vi "rsidr_core_global.vi"() -> ()   [LabVIEW 2015, in "Rohde&Schwarz CMXP NR FR2 Measurement.lvlib"] (continued)
  in  "Range Tables":T3(array[cluster])=[{"Name"="rsCmxpNrFr2M_rngInputConnector", "Type"=enum."Discrete", "Entries"=[{"Name"="RF1COM", "Discrete or Min"=1.0, "Max"=0.0, "Coerced"=0.0, "Command"="\"P1.RRH.RF1\""}, {"Name"="RF2COM", "Discrete or Min"=2.0, "Max"=0.0, "Coerced"=0.0, "Command"="\"P1.RRH.RF2\""}, {"Name"="RF3COM", "Discrete or Min"=3.0, "Max"=0.0, "Coerced"=0.0, "Command"="\"P2.RRH.RF1\""}, {"Name"="RF4COM", "Discrete or Min"=4.0, "Max"=0.0, "Coerced"=0.0, "Command"="\"P2.RRH.RF2\""}, {"Name"="RF5COM", "Discrete or Min"=5.0, "Max"=0.0, "Coerced"=0.0, "Command"="\"P3.RRH.RF1\""}, {"Name"="RF6COM", "Discrete or Min"=6.0, "Max"=0.0, "Coerced"=0.0, "Command"="\"P3.RRH.RF2\""}, {"Name"="IF1IN", "Discrete or Min"=7.0, "Max"=0.0, "Coerced"=0.0, "Command"="\"P1.IFIn\""}, {"Name"="IF2IN", "Discrete or Min"=8.0, "Max"=0.0, "Coerced"=0.0, "Command"="\"P2.IFIn\""}, {"Name"="IF3IN", "Discrete or Min"=9.0, "Max"=0.0, "Coerced"=0.0, "Command"="\"P3.IFIn\""}]}, {"Name"="rsCmxpNrFr2M_rngExtAtt", "Type"=enum."Range", "Entries"=[{"Name"="", "Discrete or Min"=-50.0, "Max"=90.0, "Coerced"=0.0, "Command"=""}]}, {"Name"="rsCmxpNrFr2M_rngRepMode", "Type"=enum."Discrete", "Entries"=[{"Name"="Single shot measurement", "Discrete or Min"=0.0, "Max"=0.0, "Coerced"=0.0, "Command"="SING"}, {"Name"="Continuous measurement", "Discrete or Min"=1.0, "Max"=0.0, "Coerced"=0.0, "Command"="CONT"}]}, {"Name"="rsCmxpNrFr2M_rngStatCount", "Type"=enum."Range", "Entries"=[{"Name"="", "Discrete or Min"=1.0, "Max"=1000.0, "Coerced"=0.0, "Command"=""}]}, {"Name"="rsCmxpNrFr2M_rngTrigThreshold", "Type"=enum."Range", "Entries"=[{"Name"="", "Discrete or Min"=-50.0, "Max"=0.0, "Coerced"=0.0, "Command"=""}]}, {"Name"="rsCmxpNrFr2M_rngStopCondition", "Type"=enum."Discrete", "Entries"=[{"Name"="None", "Discrete or Min"=0.0, "Max"=0.0, "Coerced"=0.0, "Command"="NONE"}, {"Name"="Limit Failure", "Discrete or Min"=1.0, "Max"=0.0, "Coerced"=0.0, "Command"="SLF"}]}, {"Name"="rsCmxpNrFr2M_rngTrigSlope", "Type"=enum."Discrete", "Entries"=[{"Name"="Rising edge", "Discrete or Min"=0.0, "Max"=0.0, "Coerced"=0.0, "Command"="REDG"}, {"Name"="Falling Edge", "Discrete or Min"=1.0, "Max"=0.0, "Coerced"=0.0, "Command"="FEDG"}]}, {"Name"="rsCmxpNrFr2M_rngAnalyzerMixerLevelOffset", "Type"=enum."Range", "Entries"=[{"Name"="", "Discrete or Min"=-10.0, "Max"=10.0, "Coerced"=0.0, "Command"=""}]}, {"Name"="rsCmxpNrFr2M_rngInputSignalFrequencyBand", "Type"=enum."Discrete", "Entries"=[{"Name"="Band n257", "Discrete or Min"=0.0, "Max"=0.0, "Coerced"=0.0, "Command"="B257"}, {"Name"="Band n258", "Discrete or Min"=1.0, "Max"=0.0, "Coerced"=0.0, "Command"="B258"}, {"Name"="Band n260", "Discrete or Min"=2.0, "Max"=0.0, "Coerced"=0.0, "Command"="B260"}, {"Name"="Band n261", "Discrete or Min"=3.0, "Max"=0.0, "Coerced"=0.0, "Command"="B261"}]}, {"Name"="rsCmxpNrFr2M_rngAnalyzerFrequencyOffset", "Type"=enum."Range", "Entries"=[{"Name"="", "Discrete or Min"=-100000.0, "Max"=100000.0, "Coerced"=0.0, "Command"=""}]}, {"Name"="rsCmxpNrFr2M_rngMeasurementMode", "Type"=enum."Discrete", "Entries"=[{"Name"="Normal", "Discrete or Min"=0.0, "Max"=0.0, "Coerced"=0.0, "Command"="NORM"}, {"Name"="List Mode", "Discrete or Min"=1.0, "Max"=0.0, "Coerced"=0.0, "Command"="MELM"}]}, {"Name"="rsCmxpNrFr2M_rngListBand", "Type"=enum."Discrete", "Entries"=[{"Name"="B257", "Discrete or Min"=0.0, "Max"=0.0, "Coerced"=0.0, "Command"="B257"}, {"Name"="B258", "Discrete or Min"=1.0, "Max"=0.0, "Coerced"=0.0, "Command"="B258"}, {"Name"="B260", "Discrete or Min"=2.0, "Max"=0.0, "Coerced"=0.0, "Command"="B260"}, {"Name"="B261", "Discrete or Min"=3.0, "Max"=0.0, "Coerced"=0.0, "Command"="B261"}]}, {"Name"="rsCmxpNrFr2M_rngModScheme", "Type"=enum."Discrete", "Entries"=[{"Name"="Pi/2-BPSK", "Discrete or Min"=0.0, "Max"=0.0, "Coerced"=0.0, "Command"="PHBP"}, {"Name"="QPSK", "Discrete or Min"=1.0, "Max"=0.0, "Coerced"=0.0, "Command"="QPSK"}, {"Name"="16-QAM", "Discrete or Min"=2.0, "Max"=0.0, "Coerced"=0.0, "Command"="Q16"}, {"Name"="64-QAM", "Discrete or Min"=3.0, "Max"=0.0, "Coerced"=0.0, "Command"="Q64"}, {"Name"="256-QAM", "Discrete or Min"=4.0, "Max"=0.0, "Coerced"=0.0, "Command"="Q256"}]}, {"Name"="rsCmxpNrFr2M_rngOBWLimit", "Type"=enum."Range", "Entries"=[{"Name"="", "Discrete or Min"=0.0, "Max"=400000000.0, "Coerced"=0.0, "Command"=""}]}, {"Name"="rsCmxpNrFr2M_rngPhaseComp", "Type"=enum."Discrete", "Entries"=[{"Name"="Off", "Discrete or Min"=0.0, "Max"=0.0, "Coerced"=0.0, "Command"="OFF"}, {"Name"="Carrier Freq", "Discrete or Min"=1.0, "Max"=0.0, "Coerced"=0.0, "Command"="CAF"}, {"Name"="User Defined", "Discrete or Min"=2.0, "Max"=0.0, "Coerced"=0.0, "Command"="UDEF"}]}, {"Name"="rsCmxpNrFr2M_rngPUSCHMappingType", "Type"=enum."Discrete", "Entries"=[{"Name"="A", "Discrete or Min"=0.0, "Max"=0.0, "Coerced"=0.0, "Command"="A"}, {"Name"="B", "Discrete or Min"=1.0, "Max"=0.0, "Coerced"=0.0, "Command"="B"}]}, {"Name"="rsCmxpNrFr2M_rngPhysicalCellID", "Type"=enum."Range", "Entries"=[{"Name"="", "Discrete or Min"=0.0, "Max"=1007.0, "Coerced"=0.0, "Command"=""}]}, {"Name"="rsCmxpNrFr2M_rngTypeAPosition", "Type"=enum."Range", "Entries"=[{"Name"="", "Discrete or Min"=2.0, "Max"=3.0, "Coerced"=0.0, "Command"=""}]}, {"Name"="rsCmxpNrFr2M_rngTriggerTimeout", "Type"=enum."Range", "Entries"=[{"Name"="", "Discrete or Min"=0.01, "Max"=167772.15, "Coerced"=0.0, "Command"=""}]}, {"Name"="rsCmxpNrFr2M_rngResultType", "Type"=enum."Discrete", "Entries"=[{"Name"="Current", "Discrete or Min"=0.0, "Max"=0.0, "Coerced"=0.0, "Command"="CURR"}, {"Name"="Average", "Discrete or Min"=1.0, "Max"=0.0, "Coerced"=0.0, "Command"="AVER"}, {"Name"="Extreme", "Discrete or Min"=2.0, "Max"=0.0, "Coerced"=0.0, "Command"="EXTR"}, {"Name"="Standard Deviation", "Discrete or Min"=3.0, "Max"=0.0, "Coerced"=0.0, "Command"="SDEV"}, {"Name"="Maximum", "Discrete or Min"=4.0, "Max"=0.0, "Coerced"=0.0, "Command"="MAX"}, {"Name"="Minimum", "Discrete or Min"=5.0, "Max"=0.0, "Coerced"=0.0, "Command"="MIN"}]}, {"Name"="rsCmxpNrFr2M_rngWindowPosition", "Type"=enum."Discrete", "Entries"=[{"Name"="Low", "Discrete or Min"=0.0, "Max"=0.0, "Coerced"=0.0, "Command"="LOW"}, {"Name"="High", "Discrete or Min"=1.0, "Max"=0.0, "Coerced"=0.0, "Command"="HIGH"}]}, {"Name"="rsCmxpNrFr2M_rngPosNeg", "Type"=enum."Discrete", "Entries"=[{"Name"="Negative", "Discrete or Min"=0.0, "Max"=0.0, "Coerced"=0.0, "Command"="NEG"}, {"Name"="Positive", "Discrete or Min"=1.0, "Max"=0.0, "Coerced"=0.0, "Command"="POS"}]}, {"Name"="rsCmxpNrFr2M_rngMaxMin", "Type"=enum."Discrete", "Entries"=[{"Name"="Minimum", "Discrete or Min"=0.0, "Max"=0.0, "Coerced"=0.0, "Command"="MIN"}, {"Name"="Maximum", "Discrete or Min"=1.0, "Max"=0.0, "Coerced"=0.0, "Command"="MAX"}]}, {"Name"="rsCmxpNrFr2M_rngLowHigh", "Type"=enum."Discrete", "Entries"=[{"Name"="Low", "Discrete or Min"=0.0, "Max"=0.0, "Coerced"=0.0, "Command"="LOW"}, {"Name"="High", "Discrete or Min"=1.0, "Max"=0.0, "Coerced"=0.0, "Command"="HIGH"}]}, {"Name"="rsCmxpNrFr2M_rngPeriodicity", "Type"=enum."Discrete", "Entries"=[{"Name"="0.5 ms", "Discrete or Min"=0.0, "Max"=0.0, "Coerced"=0.0, "Command"="MS05"}, {"Name"="0.625 ms", "Discrete or Min"=1.0, "Max"=0.0, "Coerced"=0.0, "Command"="MS0625"}, {"Name"="1 ms", "Discrete or Min"=2.0, "Max"=0.0, "Coerced"=0.0, "Command"="MS1"}, {"Name"="1.25 ms", "Discrete or Min"=3.0, "Max"=0.0, "Coerced"=0.0, "Command"="MS125"}, {"Name"="2 ms", "Discrete or Min"=4.0, "Max"=0.0, "Coerced"=0.0, "Command"="MS2"}, {"Name"="2.5 ms", "Discrete or Min"=5.0, "Max"=0.0, "Coerced"=0.0, "Command"="MS25"}, {"Name"="5 ms", "Discrete or Min"=6.0, "Max"=0.0, "Coerced"=0.0, "Command"="MS5"}, {"Name"="10 ms", "Discrete or Min"=7.0, "Max"=0.0, "Coerced"=0.0, "Command"="MS10"}]}, {"Name"="rsCmxpNrFr2M_rngSubcarrierSpacing", "Type"=enum."Discrete", "Entries"=[{"Name"="60 kHz", "Discrete or Min"=0.0, "Max"=0.0, "Coerced"=0.0, "Command"="S60K"}, {"Name"="120 kHz", "Discrete or Min"=1.0, "Max"=0.0, "Coerced"=0.0, "Command"="S120"}]}, {"Name"="rsCmxpNrFr2M_rngChannelBandwidth", "Type"=enum."Discrete", "Entries"=[{"Name"="50 MHz", "Discrete or Min"=0.0, "Max"=0.0, "Coerced"=0.0, "Command"="B050"}, {"Name"="100 MHz", "Discrete or Min"=1.0, "Max"=0.0, "Coerced"=0.0, "Command"="B100"}, {"Name"="200 MHz", "Discrete or Min"=2.0, "Max"=0.0, "Coerced"=0.0, "Command"="B200"}, {"Name"="400 MHz", "Discrete or Min"=3.0, "Max"=0.0, "Coerced"=0.0, "Command"="B400"}]}, {"Name"="rsCmxpNrFr2M_rngDMRSSequenceGenerationUsedID", "Type"=enum."Discrete", "Entries"=[{"Name"="Cell ID Used", "Discrete or Min"=0.0, "Max"=0.0, "Coerced"=0.0, "Command"="CID"}, {"Name"="DMRS ID Used", "Discrete or Min"=1.0, "Max"=0.0, "Coerced"=0.0, "Command"="DMRS"}]}, {"Name"="rsCmxpNrFr2M_rngBandwidthFrequency", "Type"=enum."Discrete", "Entries"=[{"Name"="50 MHz", "Discrete or Min"=0.0, "Max"=0.0, "Coerced"=0.0, "Command"="50"}, {"Name"="100 MHz", "Discrete or Min"=1.0, "Max"=0.0, "Coerced"=0.0, "Command"="100"}, {"Name"="200 MHz", "Discrete or Min"=2.0, "Max"=0.0, "Coerced"=0.0, "Command"="200"}, {"Name"="400 MHz", "Discrete or Min"=3.0, "Max"=0.0, "Coerced"=0.0, "Command"="400"}]}, {"Name"="rsCmxpNrFr2M_rngMultiEvalMeasurementSpectrumMeasFilter", "Type"=enum."Discrete", "Entries"=[{"Name"="Bandpass", "Discrete or Min"=0.0, "Max"=0.0, "Coerced"=0.0, "Command"="BAND"}, {"Name"="Gauss", "Discrete or Min"=1.0, "Max"=0.0, "Coerced"=0.0, "Command"="GAUS"}]}, {"Name"="rsCmxpNrFr2M_rngMultiEvalMeasurementTriggerDelay", "Type"=enum."Range", "Entries"=[{"Name"="", "Discrete or Min"=-0.00025, "Max"=0.00025, "Coerced"=0.0, "Command"=""}]}, {"Name"="rsCmxpNrFr2M_rngMultiEvalMeasurementMinimumTriggerGap", "Type"=enum."Range", "Entries"=[{"Name"="", "Discrete or Min"=0.0, "Max"=0.001, "Coerced"=0.0, "Command"=""}]}, {"Name"="rsCmxpNrFr2M_rngRetriggerFlag", "Type"=enum."Discrete", "Entries"=[{"Name"="Off", "Discrete or Min"=0.0, "Max"=0.0, "Coerced"=0.0, "Command"="OFF"}, {"Name"="On", "Discrete or Min"=1.0, "Max"=0.0, "Coerced"=0.0, "Command"="ON"}, {"Name"="IF Power", "Discrete or Min"=2.0, "Max"=0.0, "Coerced"=0.0, "Command"="IFP"}]}, {"Name"="rsCmxpNrFr2M_rngLimitEnabled", "Type"=enum."Discrete", "Entries"=[{"Name"="Off", "Discrete or Min"=0.0, "Max"=0.0, "Coerced"=0.0, "Command"="OFF"}, {"Name"="On", "Discrete or Min"=1.0, "Max"=0.0, "Coerced"=0.0, "Command"="ON"}, {"Name"="Value", "Discrete or Min"=2.0, "Max"=0.0, "Coerced"=0.0, "Command"="VAL"}]}, {"Name"="rsCmxpNrFr2M_rngMultiEvalMeasurementLimitACLR", "Type"=enum."Discrete", "Entries"=[{"Name"="Band n257, n258, n261", "Discrete or Min"=1.0, "Max"=0.0, "Coerced"=0.0, "Command"="1"}, {"Name"="Bands n260", "Discrete or Min"=2.0, "Max"=0.0, "Coerced"=0.0, "Command"="2"}]}, {"Name"="rsCmxpNrFr2M_rngUserDefFreq", "Type"=enum."Range", "Entries"=[{"Name"="", "Discrete or Min"=24250000000.0, "Max"=52600000000.0, "Coerced"=0.0, "Command"=""}]}, {"Name"="rsCmxpNrFr2M_rngDLSlots", "Type"=enum."Range", "Entries"=[{"Name"="", "Discrete or Min"=0.0, "Max"=78.0, "Coerced"=0.0, "Command"=""}]}, {"Name"="rsCmxpNrFr2M_rngDLSymbols", "Type"=enum."Range", "Entries"=[{"Name"="", "Discrete or Min"=0.0, "Max"=14.0, "Coerced"=0.0, "Command"=""}]}, {"Name"="rsCmxpNrFr2M_rngULSlots", "Type"=enum."Range", "Entries"=[{"Name"="", "Discrete or Min"=0.0, "Max"=80.0, "Coerced"=0.0, "Command"=""}]}, {"Name"="rsCmxpNrFr2M_rngULSymbols", "Type"=enum."Range", "Entries"=[{"Name"="", "Discrete or Min"=0.0, "Max"=14.0, "Coerced"=0.0, "Command"=""}]}, {"Name"="rsCmxpNrFr2M_rngBandwidthPart", "Type"=enum."Discrete", "Entries"=[{"Name"="BWP0", "Discrete or Min"=0.0, "Max"=0.0, "Coerced"=0.0, "Command"="BWP0"}]}, {"Name"="rsCmxpNrFr2M_rngCyclicPrefix", "Type"=enum."Discrete", "Entries"=[{"Name"="Normal", "Discrete or Min"=0.0, "Max"=0.0, "Coerced"=0.0, "Command"="NORM"}]}, {"Name"="rsCmxpNrFr2M_rngNumberOfRBs", "Type"=enum."Range", "Entries"=[{"Name"="", "Discrete or Min"=11.0, "Max"=264.0, "Coerced"=0.0, "Command"=""}]}, {"Name"="rsCmxpNrFr2M_rngStartRB", "Type"=enum."Range", "Entries"=[{"Name"="", "Discrete or Min"=0.0, "Max"=253.0, "Coerced"=0.0, "Command"=""}]}, {"Name"="rsCmxpNrFr2M_rngDMRSConfigType", "Type"=enum."Range", "Entries"=[{"Name"="", "Discrete or Min"=1.0, "Max"=2.0, "Coerced"=0.0, "Command"=""}]}, {"Name"="rsCmxpNrFr2M_rngDMRSAdditionalPosition", "Type"=enum."Range", "Entries"=[{"Name"="", "Discrete or Min"=0.0, "Max"=3.0, "Coerced"=0.0, "Command"=""}]}, {"Name"="rsCmxpNrFr2M_rngDMRSMaxLength", "Type"=enum."Range", "Entries"=[{"Name"="", "Discrete or Min"=1.0, "Max"=1.0, "Coerced"=0.0, "Command"=""}]}, {"Name"="rsCmxpNrFr2M_rngPUSCHAllocatedOFMDSymbols", "Type"=enum."Range", "Entries"=[{"Name"="", "Discrete or Min"=4.0, "Max"=14.0, "Coerced"=0.0, "Command"=""}]}, {"Name"="rsCmxpNrFr2M_rngPUSCHAllocationStartSymbolA", "Type"=enum."Range", "Entries"=[{"Name"="", "Discrete or Min"=0.0, "Max"=0.0, "Coerced"=0.0, "Command"=""}]}, {"Name"="rsCmxpNrFr2M_rngPUSCHAllocationStartSymbolB", "Type"=enum."Range", "Entries"=[{"Name"="", "Discrete or Min"=0.0, "Max"=10.0, "Coerced"=0.0, "Command"=""}]}, {"Name"="rsCmxpNrFr2M_rngPUSCHAllocatedUploadRBs", "Type"=enum."Range", "Entries"=[{"Name"="", "Discrete or Min"=1.0, "Max"=264.0, "Coerced"=0.0, "Command"=""}]}, {"Name"="rsCmxpNrFr2M_rngPUSCHAllocationStartRB", "Type"=enum."Range", "Entries"=[{"Name"="", "Discrete or Min"=0.0, "Max"=263.0, "Coerced"=0.0, "Command"=""}]}, {"Name"="rsCmxpNrFr2M_rngPUSCHAllocationCDMGroups", "Type"=enum."Range", "Entries"=[{"Name"="", "Discrete or Min"=1.0, "Max"=3.0, "Coerced"=0.0, "Command"=""}]}, {"Name"="rsCmxpNrFr2M_rngPUSCHAllocationRelativeDMRSPower", "Type"=enum."Range", "Entries"=[{"Name"="", "Discrete or Min"=-10.0, "Max"=10.0, "Coerced"=0.0, "Command"=""}]}, {"Name"="rsCmxpNrFr2M_rngDMRSAntennaPort", "Type"=enum."Range", "Entries"=[{"Name"="", "Discrete or Min"=0.0, "Max"=1.0, "Coerced"=0.0, "Command"=""}]}, {"Name"="rsCmxpNrFr2M_rng16Bits", "Type"=enum."Range", "Entries"=[{"Name"="", "Discrete or Min"=0.0, "Max"=65535.0, "Coerced"=0.0, "Command"=""}]}, {"Name"="rsCmxpNrFr2M_rngDMRSSequenceGenerationNSCID", "Type"=enum."Range", "Entries"=[{"Name"="", "Discrete or Min"=0.0, "Max"=1.0, "Coerced"=0.0, "Command"=""}]}, {"Name"="rsCmxpNrFr2M_rngOFMDSymbol", "Type"=enum."Range", "Entries"=[{"Name"="", "Discrete or Min"=0.0, "Max"=13.0, "Coerced"=0.0, "Command"=""}]}, {"Name"="rsCmxpNrFr2M_rngListRangeStartIndex", "Type"=enum."Range", "Entries"=[{"Name"="", "Discrete or Min"=1.0, "Max"=2000.0, "Coerced"=0.0, "Command"=""}]}, {"Name"="rsCmxpNrFr2M_rngListRangeNoOfSegments", "Type"=enum."Range", "Entries"=[{"Name"="", "Discrete or Min"=1.0, "Max"=1000.0, "Coerced"=0.0, "Command"=""}]}, {"Name"="rsCmxpNrFr2M_rngListSegmentLength", "Type"=enum."Range", "Entries"=[{"Name"="", "Discrete or Min"=1.0, "Max"=1000.0, "Coerced"=0.0, "Command"=""}]}, {"Name"="rsCmxpNrFr2M_rngtListSegmentEvaluationOffset", "Type"=enum."Range", "Entries"=[{"Name"="", "Discrete or Min"=0.0, "Max"=1000.0, "Coerced"=0.0, "Command"=""}]}, {"Name"="rsCmxpNrFr2M_rngMeasurementMainState", "Type"=enum."Discrete", "Entries"=[{"Name"="Off", "Discrete or Min"=0.0, "Max"=0.0, "Coerced"=0.0, "Command"="OFF"}, {"Name"="Running", "Discrete or Min"=1.0, "Max"=0.0, "Coerced"=0.0, "Command"="RUN"}, {"Name"="Ready", "Discrete or Min"=2.0, "Max"=0.0, "Coerced"=0.0, "Command"="RDY"}]}, {"Name"="rsCmxpNrFr2M_rngtMeasurementSyncState", "Type"=enum."Discrete", "Entries"=[{"Name"="Pending", "Discrete or Min"=0.0, "Max"=0.0, "Coerced"=0.0, "Command"="PEND"}, {"Name"="Adjusted", "Discrete or Min"=1.0, "Max"=0.0, "Coerced"=0.0, "Command"="ADJ"}, {"Name"="Invalid", "Discrete or Min"=2.0, "Max"=0.0, "Coerced"=0.0, "Command"="INV"}]}, {"Name"="rsCmxpNrFr2M_rngMeasurementResourceState", "Type"=enum."Discrete", "Entries"=[{"Name"="Queued", "Discrete or Min"=0.0, "Max"=0.0, "Coerced"=0.0, "Command"="QUE"}, {"Name"="Active", "Discrete or Min"=1.0, "Max"=0.0, "Coerced"=0.0, "Command"="ACT"}, {"Name"="Invalid", "Discrete or Min"=2.0, "Max"=0.0, "Coerced"=0.0, "Command"="INV"}]}, {"Name"="rsCmxpNrFr2M_rngMeasurementLimitIQOffset", "Type"=enum."Range", "Entries"=[{"Name"="", "Discrete or Min"=-256.0, "Max"=256.0, "Coerced"=0.0, "Command"=""}]}, {"Name"="rsCmxpNrFr2M_rngMeasurementLimitInbandMin", "Type"=enum."Range", "Entries"=[{"Name"="", "Discrete or Min"=-256.0, "Max"=256.0, "Coerced"=0.0, "Command"=""}]}, {"Name"="rsCmxpNrFr2M_rngMeasurementLimitInbandRBPower", "Type"=enum."Range", "Entries"=[{"Name"="", "Discrete or Min"=-256.0, "Max"=256.0, "Coerced"=0.0, "Command"=""}]}, {"Name"="rsCmxpNrFr2M_rngMeasurementLimitInbandIQImage", "Type"=enum."Range", "Entries"=[{"Name"="", "Discrete or Min"=-256.0, "Max"=256.0, "Coerced"=0.0, "Command"=""}]}, {"Name"="rsCmxpNrFr2M_rngPercent", "Type"=enum."Range", "Entries"=[{"Name"="", "Discrete or Min"=0.0, "Max"=100.0, "Coerced"=0.0, "Command"=""}]}, {"Name"="rsCmxpNrFr2M_rnglMeasuremenFlatnessRange", "Type"=enum."Range", "Entries"=[{"Name"="", "Discrete or Min"=-256.0, "Max"=256.0, "Coerced"=0.0, "Command"=""}]}, {"Name"="rsCmxpNrFr2M_rngMeasurementFlatnessMaxMin", "Type"=enum."Range", "Entries"=[{"Name"="", "Discrete or Min"=-256.0, "Max"=256.0, "Coerced"=0.0, "Command"=""}]}, {"Name"="rsCmxpNrFr2M_rngMeasurementEmissionMaskFreq", "Type"=enum."Range", "Entries"=[{"Name"="", "Discrete or Min"=0.0, "Max"=405000000.0, "Coerced"=0.0, "Command"=""}]}, {"Name"="rsCmxpNrFr2M_rngMeasurementEmissionMaskLevel", "Type"=enum."Range", "Entries"=[{"Name"="", "Discrete or Min"=-256.0, "Max"=256.0, "Coerced"=0.0, "Command"=""}]}, {"Name"="rsCmxpNrFr2M_rngMultiEvalMeasurementEmissionMaskRBW", "Type"=enum."Discrete", "Entries"=[{"Name"="1 MHz", "Discrete or Min"=0.0, "Max"=0.0, "Coerced"=0.0, "Command"="M1"}]}, {"Name"="rsCmxpNrFr2M_rngMeasurementEmissionMaskTestTolerance", "Type"=enum."Range", "Entries"=[{"Name"="", "Discrete or Min"=-10.0, "Max"=10.0, "Coerced"=0.0, "Command"=""}]}, {"Name"="rsCmxpNrFr2M_rngMeasurementACLRTestTolerance", "Type"=enum."Range", "Entries"=[{"Name"="", "Discrete or Min"=-10.0, "Max"=10.0, "Coerced"=0.0, "Command"=""}]}, {"Name"="rsCmxpNrFr2M_rngLimitCheckResults", "Type"=enum."Discrete", "Entries"=[{"Name"="Pass", "Discrete or Min"=0.0, "Max"=0.0, "Coerced"=0.0, "Command"="OK"}, {"Name"="Failed Upper", "Discrete or Min"=1.0, "Max"=0.0, "Coerced"=0.0, "Command"="ULEU"}, {"Name"="Failed Lower", "Discrete or Min"=2.0, "Max"=0.0, "Coerced"=0.0, "Command"="ULEL"}, {"Name"="Overflow", "Discrete or Min"=3.0, "Max"=0.0, "Coerced"=0.0, "Command"="OFL"}, {"Name"="Underflow", "Discrete or Min"=4.0, "Max"=0.0, "Coerced"=0.0, "Command"="UFL"}, {"Name"="Invalid", "Discrete or Min"=5.0, "Max"=0.0, "Coerced"=0.0, "Command"="INV"}, {"Name"="Not A Value", "Discrete or Min"=6.0, "Max"=0.0, "Coerced"=0.0, "Command"="NAV"}]}]
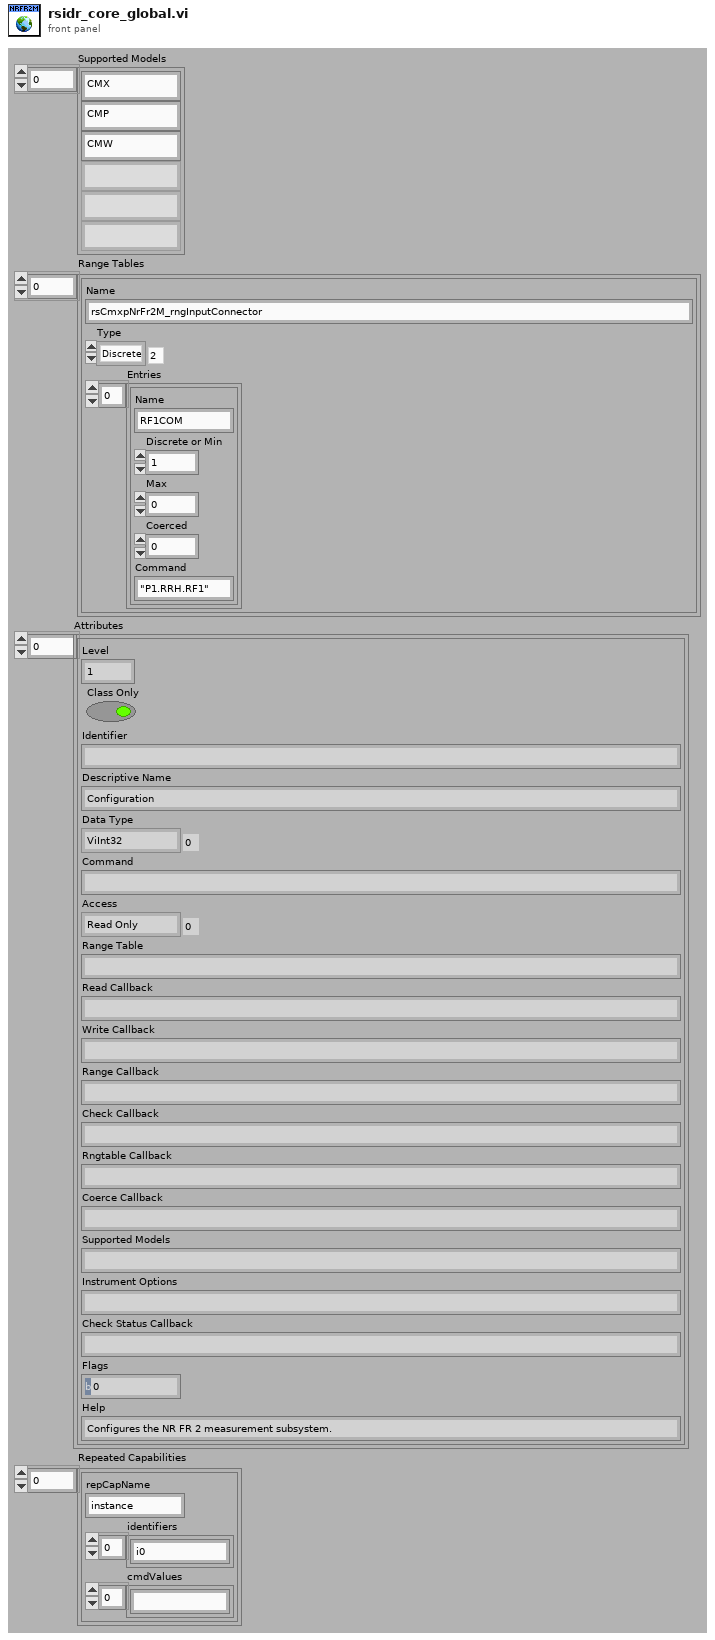
[diagram p1: front panel]
types:
  T1 = cluster{"Level":i32, "Class Only":bool, "Identifier":string, "Descriptive Name":string, "Data Type":enum16{"ViInt32", "ViReal64", "ViString", "ViBoolean", "None", "ViInt64", "RawString"}, "Command":string, "Access":enum16{"Read Only", "Write Only", "Read/Write"}, "Range Table":string, "Read Callback":string, "Write Callback":string, "Range Callback":string, "Check Callback":string, "Rngtable Callback":string, "Coerce Callback":string, "Supported Models":string, "Instrument Options":string, "Check Status Callback":string, "Flags":i32, "Help":string}[]
  T2 = cluster{"repCapName":string, "identifiers":string[], "cmdValues":string[]}[]
  T3 = cluster{"Name":string, "Type":enum16{"Range", "Coerced", "Discrete"}, "Entries":cluster{"Name":string, "Discrete or Min":dbl, "Max":dbl, "Coerced":dbl, "Command":string}[]}[]
diagram:
